vi "createFolderWithTimeInfo.vi"(10 "Folder to save file to":path=path "C:/Users/Frederic Schmitt/Desktop/GE/Sciospec Bioimpedance - Sinan/Sciospec ISX3v2/Data from LabVIEW") -> (3 "created path":path)   [LabVIEW 2012]
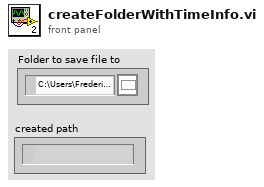
[diagram p1: front panel]
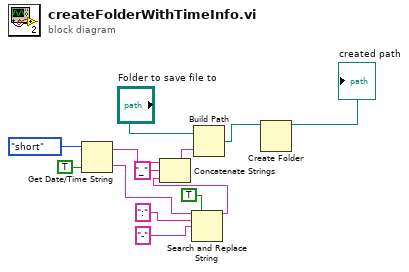
[diagram p0: block diagram]
diagram:
  n1 = Get Date/Time String(date format (0)=enum16{"short", "long", "abbreviated"}."short", want seconds? (F)=TRUE) -> (date string=w6:string, time string=w11:string)  [unwired: 1 in]
  n2 = Search and Replace String(replace all?=TRUE ("replace all? (F)"), input string=w11, search string=":" ("replace string (\"\")"), replace string="-" ("replace string (\"\")")) -> (result string=w12:string)  [unwired: 4 in, 3 out]
  n3 = Concatenate Strings(w6, "_" ("string"), w12) -> (w7:string)
  n4 = Build Path(base path="Folder to save file to", name or relative path=w7) -> (appended path=w5:path)
  n5 = Create Folder(path (use dialog)=w5) -> (created path=→"created path":path)  [unwired: 2 in, 2 out]
